vi "Dispose Kinect.vi"(3 "error in (no error)":errorcluster, 4 "Queues In":T1, 5 "References":T2) -> (0 "error out":errorcluster)   [LabVIEW 2011, in "Kinect_API.lvlib"]
uses:
  Kinect_API.lvlib
  Microsoft.Research.Kinect
  <vilib>/vision/Image Controls.llb/IMAQ Image.ctl
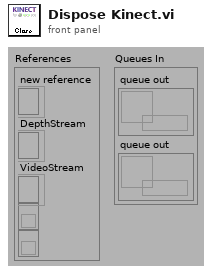
[diagram p1: front panel]
types:
  T1 = cluster{"queue out":refnum<queue>, "queue out":refnum<queue>}
  T2 = cluster{"new reference":refnum<k24>, "DepthStream":refnum<k24>, "VideoStream":refnum<k24>, "Event Callback":refnum<k27>, "Event Callback":refnum<k27>}
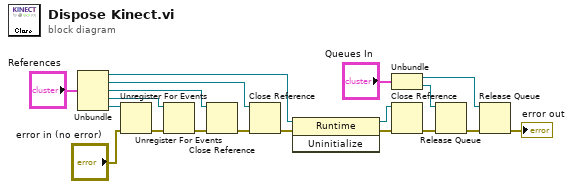
[diagram p0: block diagram]
diagram:
  n1 = Unbundle("References") -> ("new reference"=w4:refnum<k24>, "DepthStream"=w15:refnum<k24>, "VideoStream"=w14:refnum<k24>, "Event Callback"=w13:refnum<k27>, "Event Callback"=w12:refnum<k27>)
  n2 = Unregister For Events(event registration refnum=w12, error in="error in (no error)") -> (error out=w18:errorcluster)
  n3 = Unregister For Events(event registration refnum=w13, error in=w18) -> (error out=w17:errorcluster)
  n4 = Close Reference(reference=w14, error in (no error)=w17) -> (error out=w19:errorcluster)
  n5 = Close Reference(reference=w15, error in (no error)=w19) -> (error out=w3:errorcluster)
  n6 = invoke class="Runtime" method="Uninitialize"(reference=w4, error in=w3) -> (reference out=w1:refnum<k24>, error out=w2:errorcluster)  [unwired: 1 in, 1 out]
  n7 = Unbundle("Queues In") -> ("queue out"=w5:refnum<queue>, "queue out"=w6:refnum<queue>)
  n8 = Close Reference(reference=w1, error in (no error)=w2) -> (error out=w9:errorcluster)
  n9 = Release Queue(queue=w6, error in (no error)=w9) -> (error out=w8:errorcluster)  [unwired: 1 in, 2 out]
  n10 = Release Queue(queue=w5, error in (no error)=w8) -> (error out=→"error out":errorcluster)  [unwired: 1 in, 2 out]
